vi "Controllers.vi"   [LabVIEW 2018]
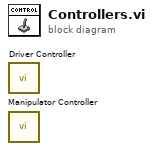
[diagram p0: block diagram]
diagram:
  n1 = call "Driver Controller.vi"() -> ()  [unwired: 12 in]
  n2 = call "Manipulator Controller.vi"() -> ()  [unwired: 12 in]
